vi "Recurse.vi"(6 "Teller":T1 {"Time" format="%<%x %.3X>T"}, 7 "Actor in":refnum<class "Actor.lvclass">, 8 "Error in":errorcluster) -> (0 "Error out":errorcluster, 5 "Actor out":refnum<class "Actor.lvclass">)   [LabVIEW 2020, in "jettl.lvlib" / "Stop jettl Msg.lvlib" / "Stop.lvlib"]
uses:
  Stop.lvlib
  Actor/Actor.lvclass
  jettl.lvlib
  Stop Msg Output/Stop Msg Output.lvlib
  Relation.ctl
  Teller Metadata/Teller Metadata.lvclass
  Teller.ctl
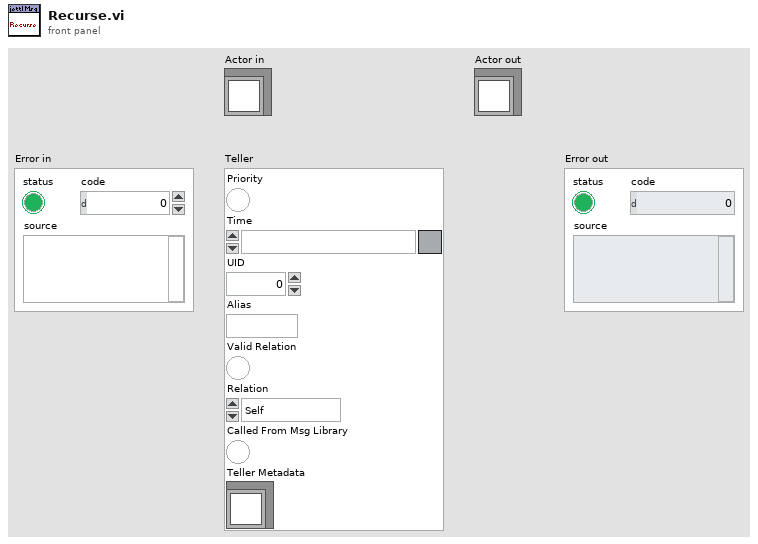
[diagram p1: front panel]
types:
  T1 = typedef "jettl.lvlib/Teller.ctl" = cluster{"Priority":bool, "Time":timestamp, "UID":i32, "Alias":string, "Valid Relation":bool, "Relation":T2, "Called From Msg Library":bool, "Teller Metadata":refnum<class "Teller Metadata.lvclass">}
  T2 = typedef "jettl.lvlib/Relation.ctl" = enum16{"Self", "Parent", "Child"}
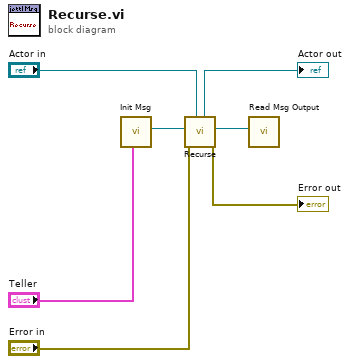
[diagram p0: block diagram]
diagram:
  n1 = call "Init Msg.vi"("Teller"="Teller") -> ("Msg"=w2:refnum<class "Msg.lvclass">)  [unwired: 10 in]
  n2 = call "Recurse.vi"("Actor in"="Actor in", "Error in"="Error in", "Msg"=w2) -> ("Error out"=→"Error out":errorcluster, "Msg Output"=w3:refnum<class "Msg Output.lvclass">, "Actor out"=→"Actor out":refnum<class "Actor.lvclass">)  [unwired: 6 in]
  n3 = call "Read Msg Output.vi"("Msg Output"=w3) -> ()  [unwired: 11 in]
